vi "Main_Host Config GBL.vi"() -> ()   [LabVIEW 2019]
doc: "JSMA Project Wizard 0.2.0.11\nRob Humfeld - JET Engineering\nCopyright (c) 2020, JET Engineering"
panel:
  out "is EXE?":bool
  in  "Host User Files Folder":path=path "../User Files"
  in  "Host Temp Files Folder":path=path "../Temp Files"
  in  "Host Config Files Folder":path=path "Config Files_Host"
  # "These Path default values are defined relative to the Software folder"
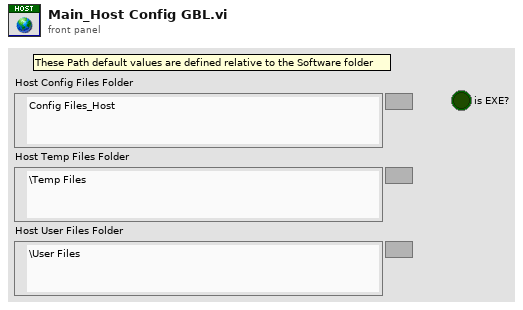
[diagram p1: front panel]
diagram:
